vi "FPGAController_v4.vi"() -> ()   [LabVIEW 2015]
uses:
  <vilib>/Utility/miscctls.llb/LVPointTypeDef.ctl
  <vilib>/FPGAPlugInAG/PXIe-7971R/niLvFpga_Open_PXIe-7971R.vi
  <vilib>/Utility/error.llb/Error Cluster From Error Code.vi
  <vilib>/rvi/errors/niLvFpgaAdjustHostInterfaceError.vi
  <userlib>/_OpenG.lib/comparison/comparison.llb/DBL Changed__ogtk.vi
  <userlib>/_OpenG.lib/file/file.llb/Strip Path Extension - Path__ogtk.vi
  <userlib>/_OpenG.lib/comparison/comparison.llb/Boolean Changed__ogtk.vi
  <vilib>/addons/database/Connection.llb/Conn Execute.vi
  <vilib>/addons/database/Recordset.llb/Rec Fetch Recordset Data (R).vi
  <vilib>/addons/database/Recordset.llb/Rec Destroy - Connection.vi
  <vilib>/FPGAPlugInAG/PXIe-7971R/niLvFpga_Close_PXIe-7971R.vi
  <vilib>/rvi/interface/nirviOpenFPGA/nirviOpenFPGA.xnode
  FPGA Bitfiles/FPGAnew_FPGATarget_FPGAcode5762_R0izv7IQhAo.lvbitx
  <vilib>/rvi/interface/nirviReadWriteControl/nirviReadWriteControl.xnode
  <vilib>/rvi/interface/nirviMethod/nirviMethod.xnode
  <vilib>/FPGA/interface/niFpgaViExecutionMode.ctl
  <vilib>/addons/database/_DB Variant To Data/Database Variant To Data.xnode
  <vilib>/rvi/interface/nirviCloseFPGA/nirviCloseFPGA.xnode
  <vilib>/addons/database/NI_Database_API.lvlib
  NiFpgaLv.dll
panel:
  out "Time Betwee Shots":dbl
  in  "Min. Time\nBetween Shots (s)":dbl
  in  "Rate Limiting":bool
  out "Update Threshold":bool
  in  "Auto Threshold":bool
  in  "stop":bool
  out "stopping":bool
  in  "One Shot Mode":bool
  out "High Velocity":dbl=100000.0
  out "Low Velocity":dbl=1000.0
  out "Low velocity count":i32=21000
  out "High velocity count":i32=210
  out "Filter 1 Peak":i32=295996
  out "Filter 2 Peak":i32=120664
  out "Filter 3 Peak":i32=46254
  out "Filter 4 Peak":i32=18191
  out "Filter 5 Peak":i32=13910
  out "Filter 6 Peak":i32=9863
  out "Filter 7 Peak":i32=7483
  in  "Zero Peak Values":bool
  in  "Peak-Threshold Factor":dbl=2.0
  in  "Assign Threshold":bool
  in  "Filter1 Threshold":i32=-887988
  in  "Filter2 Threshold":i32=-361992
  in  "Filter3 Threshold":i32=-138762
  in  "Filter4 Threshold":i32=-54306
  in  "Filter5 Threshold":i32=-41730
  in  "Filter6 Threshold":i32=-29358
  in  "Filter7 Threshold":i32=-21165
  out "High Charge Limit (fC)":dbl=100.0
  out "Low Charge Limit (fC)":dbl
  out "High Charge Limit":i16
  out "Low Charge Limit":i16
  out "Low Mass (kg)":dbl
  out "High Mass (kg)":dbl=inf
  out "Peletron (MV)":dbl=2.0
  in  "Run Mode":bool
  out "High Mass Limit":fxp<+,31,17>
  out "Low Mass Limit":fxp<+,31,17>
  out "error out":errorcluster
  out "Sensitivity":dbl
  out "Last Update:":timestamp
  out "Updating FPGA":bool
  in  "Delay Ring":dbl(ring)=3.15039 items=["Custom"]
  in  "Delay Value":dbl=3.0 min=0.0
  in  "Delay Name":string
  in  "Rearm Trigger":bool
  out "Armed":bool
  in  "Add Delay":bool
  in  "Raise Threshold":bool
  in  "Lower Threshold":bool
  out "Del Armed":bool
  # "Dubugging"
  # "Settings"
  # "Thresholds"
  # "Peaks"
  # "Independent Variable"
  # "Threshold 1"
  # "Peak 1"
  # "Low Vel."
  # "High Vel."
  # "Threshold 2"
  # "Peak 2"
  # "Low Q (fC)"
  # "High Q (fC)"
  # "Plate Control While Loop Counter"
  # "Threshold 3"
  # "Peak 3"
  # "Low Mass (kg)"
  # "High Q (fC)"
  # "Threshold 4"
  # "Peak 4"
  # "Sens. (V/pC)"
  # "Peletron (MV)"
  # "Current Value of Running Average"
  # "Threshold 5"
  # "Peak 5"
  # "Peak Threshold Factor"
  # "Threshold 6"
  # "Peak 6"
  # "Delay Trigger"
  # "Dist. from 2nd Det. (m)"
  # "Name"
  # "Threshold 7"
  # "Peak 7"
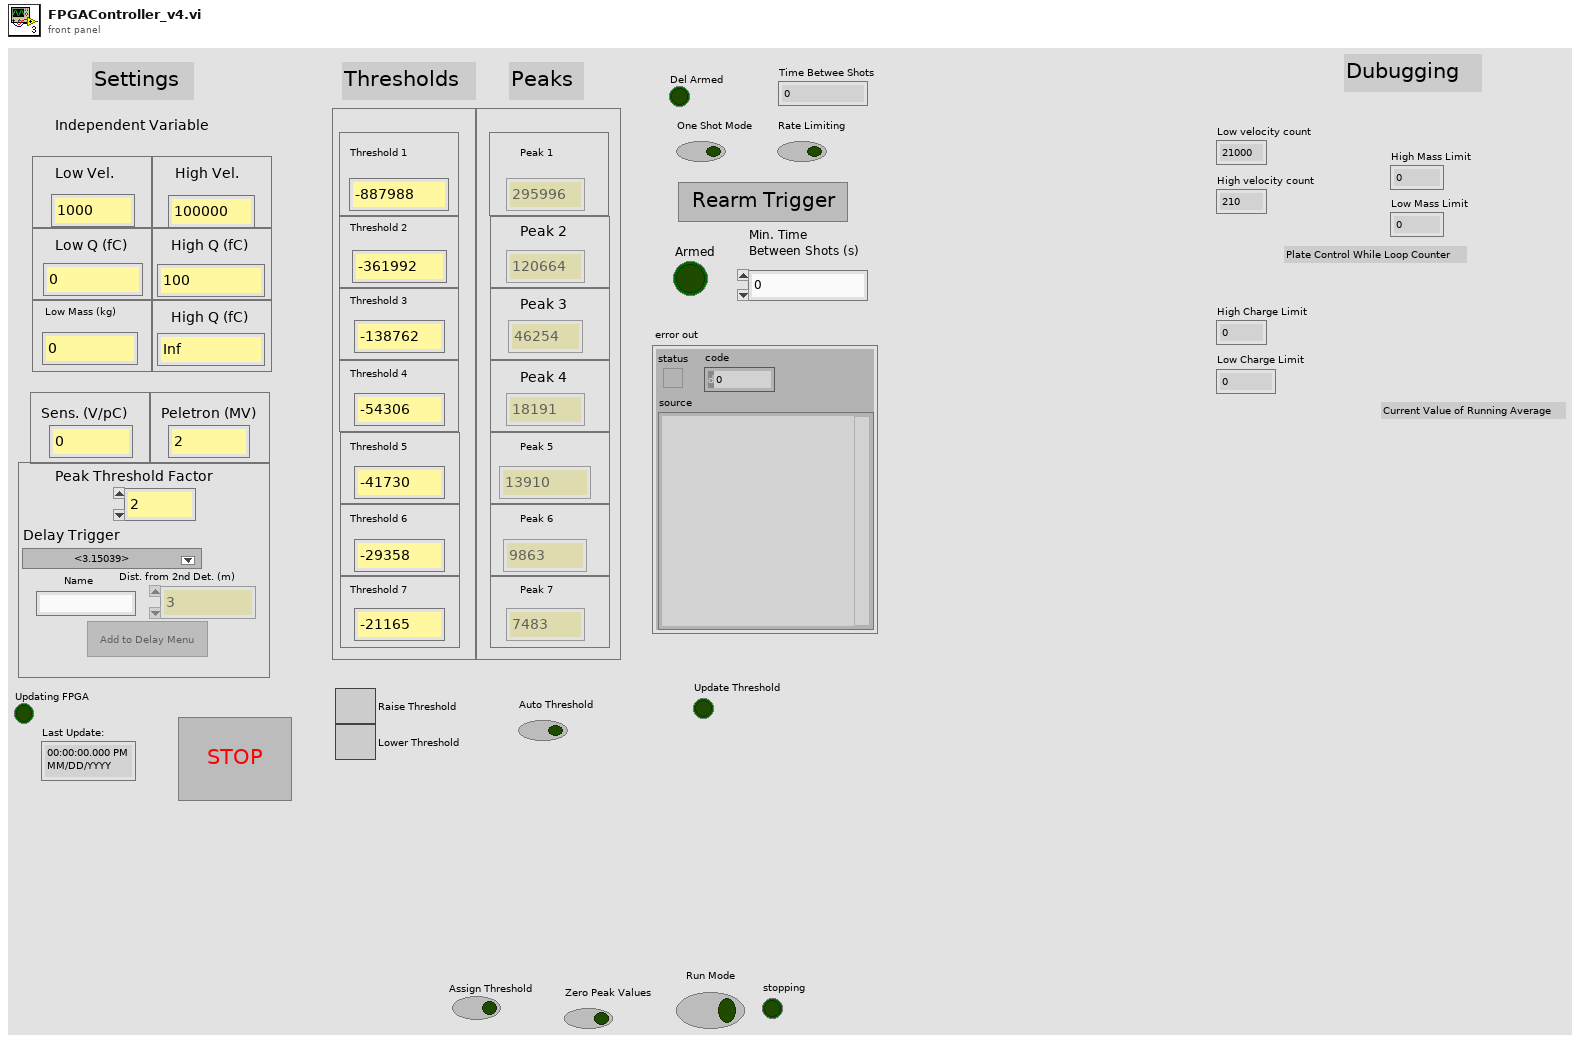
[diagram p1: front panel]
types:
  T1 = typedef "LVPointTypeDef.ctl" = cluster{"Horizontal":i16, "Vertical":i16}
  T2 = enum8{"Enabled", "Disabled", "Disabled and Grayed Out"}
  T3 = typedef "NI_Database_API.lvlib/Conn ObjectReference.ctl" = refnum<k1>
  T4 = cluster{"Filter 1 Peak":i32, "Filter 2 Peak":i32, "Filter 3 Peak":i32, "Filter 4 Peak":i32, "Filter 5 Peak":i32, "Filter 6 Peak":i32, "Filter 7 Peak":i32}
  T5 = typedef "NI_Database_API.lvlib/Rec ObjectReference.ctl" = refnum<k1>
  T6 = typedef "LVStringsAndValuesArrayTypeDef_DBL.ctl" = cluster{"String":string, "Value":dbl}[]
  T7 = cluster{"Numeric":dbl, "Numeric":dbl, "Numeric":dbl, "Numeric":dbl, "Numeric":dbl, "Numeric":dbl, i32, dbl, "Value":dbl, fxp<+,16,7>, bool}
  T8 = cluster{"Low Velocity Count":i32, "High Velocity Count":i32, "Low Charge Limit (ADC ticks)":i16, "High Charge Limit (ADC ticks)":i16, "Low Mass (ADC*cycle^2)":i64, "High Mass (ADC*cycle^2)":i64, "Mult":fxp<+,16,7>, "Mult Use?":bool}
  T9 = cluster{"Filter 1 Detector 3 Correlation":i32, "Filter 2 Detector 3 Correlation":i32, "Filter 3 Detector 3 Correlation":i32, "Filter 4 Detector 3 Correlation":i32, "Filter 5 Detector 3 Correlation":i32, "Filter 6 Detector 3 Correlation":i32, "Filter 7 Detector 3 Correlation":i32}
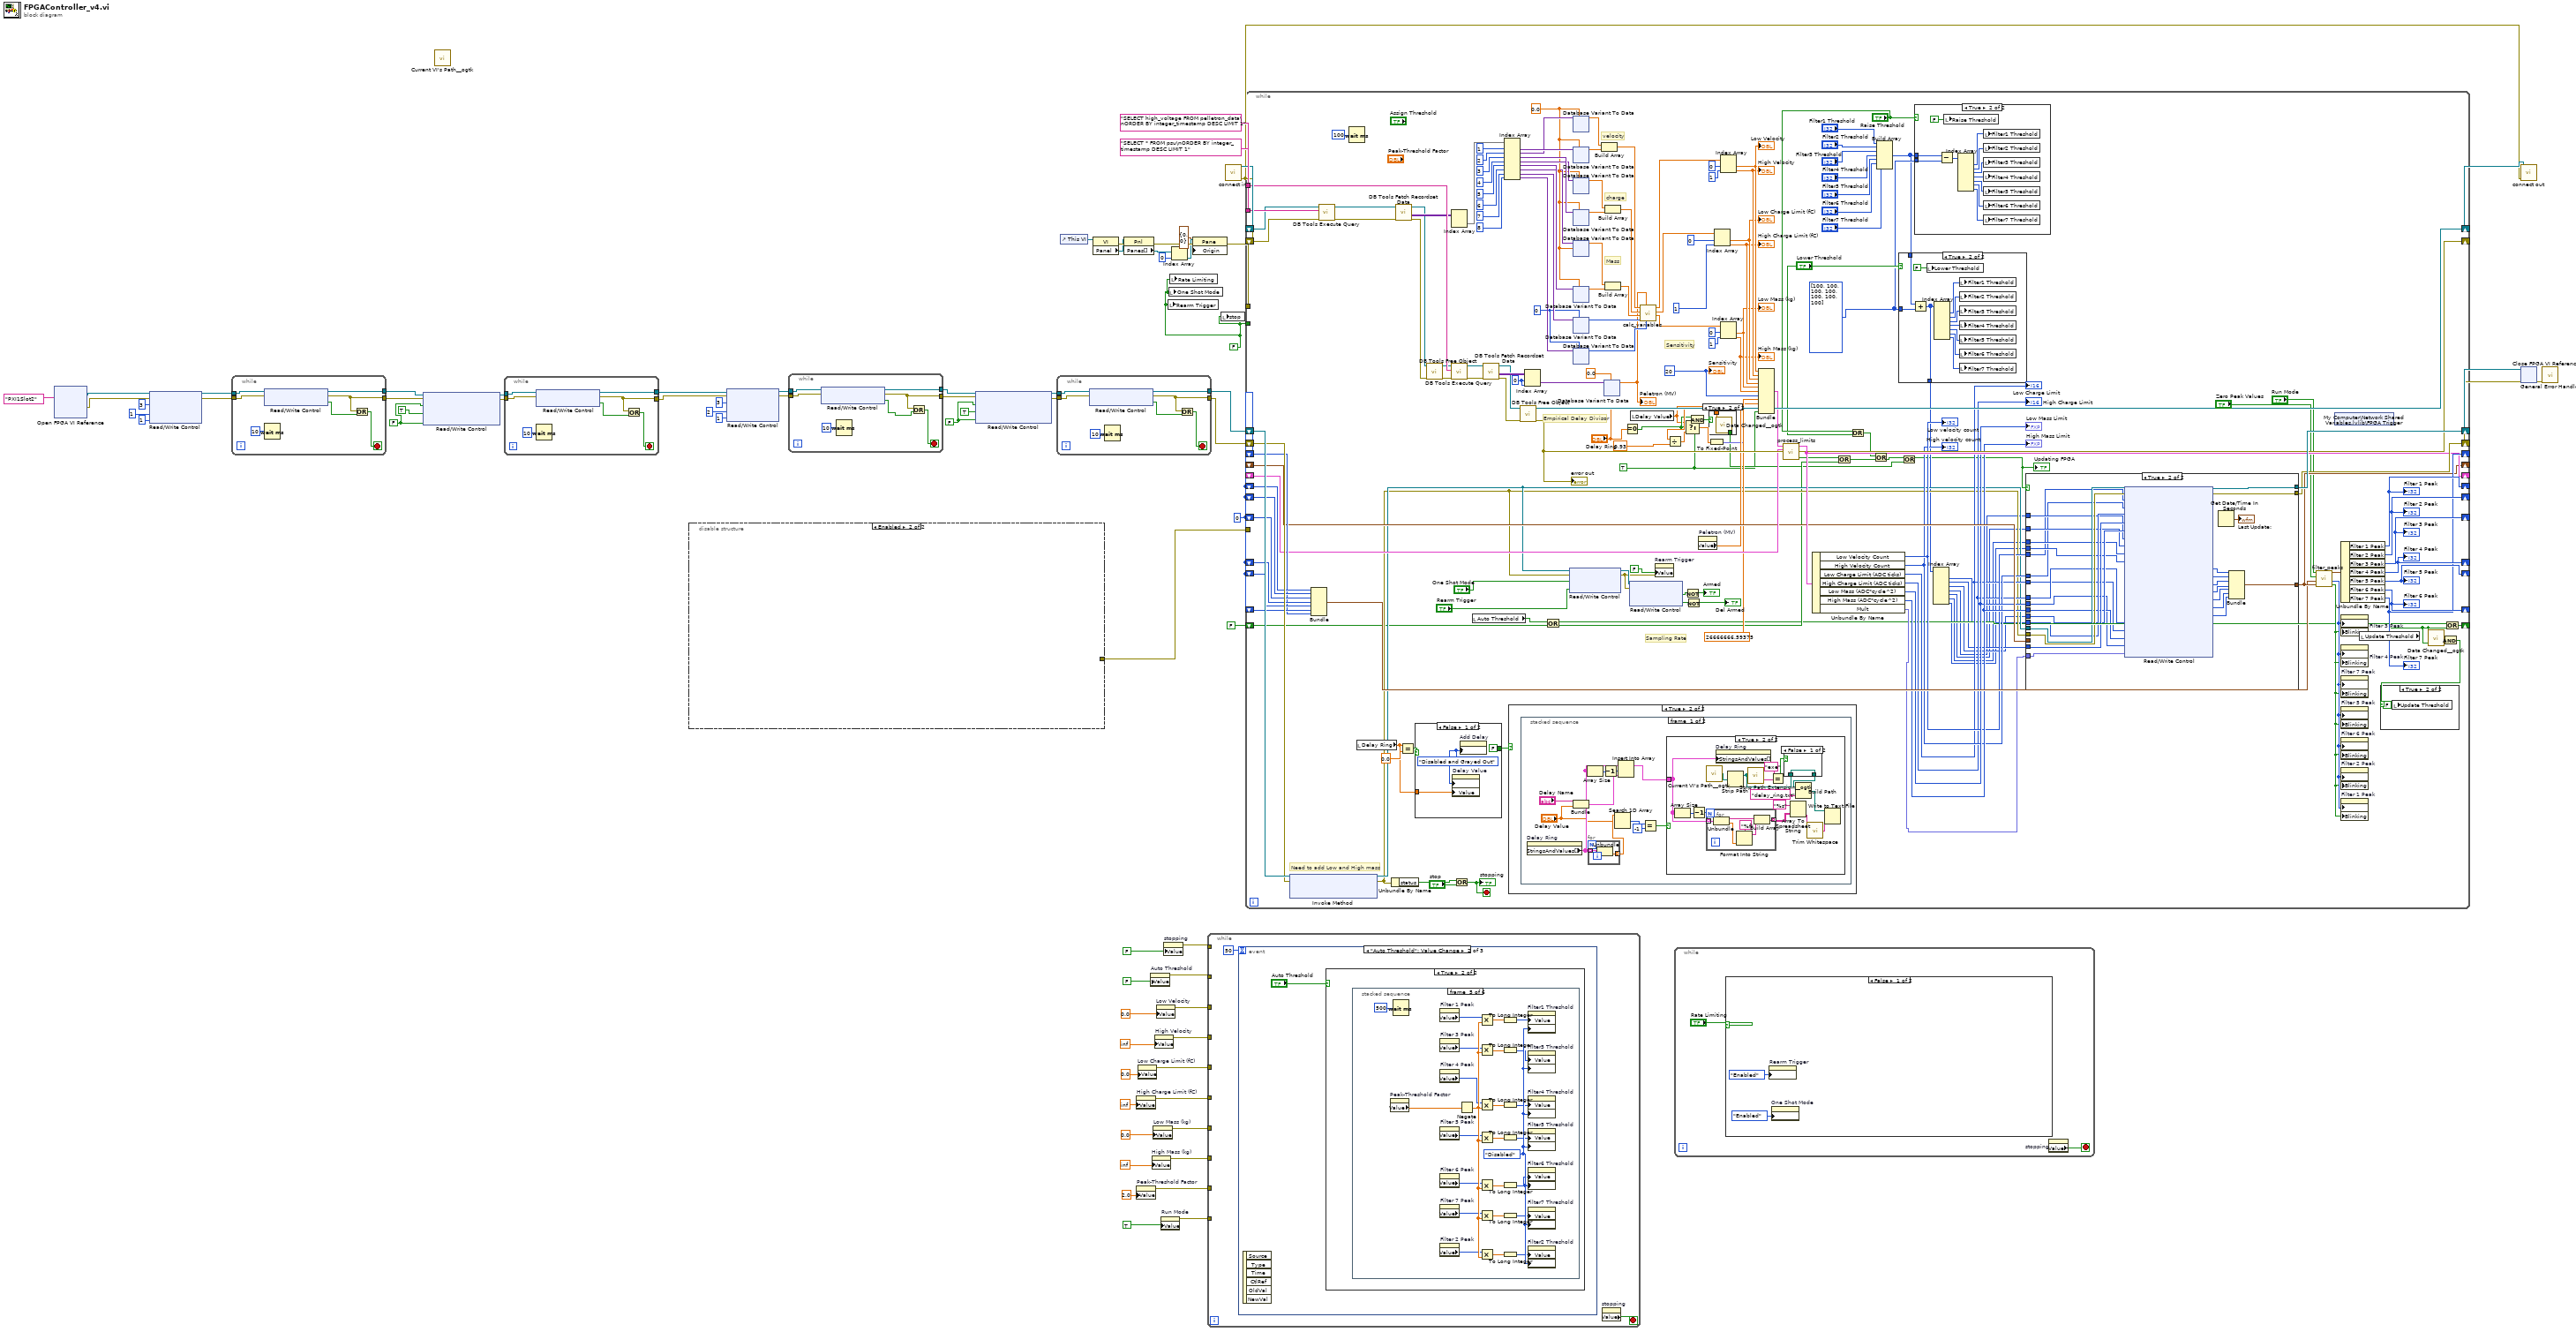
[diagram p0: block diagram]
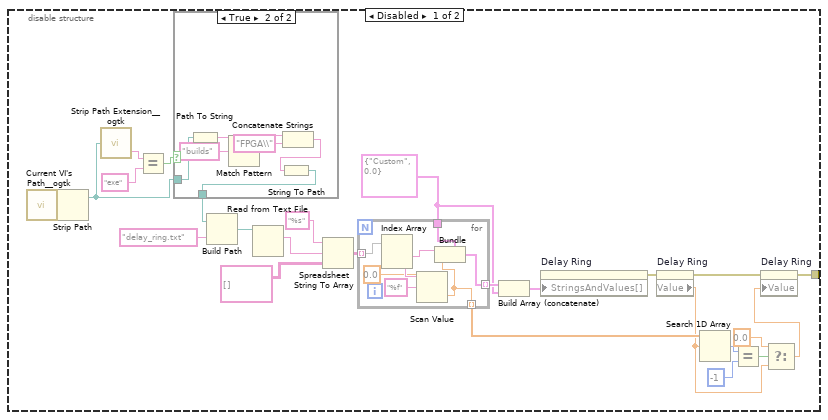
[diagram p2: hidden frame]
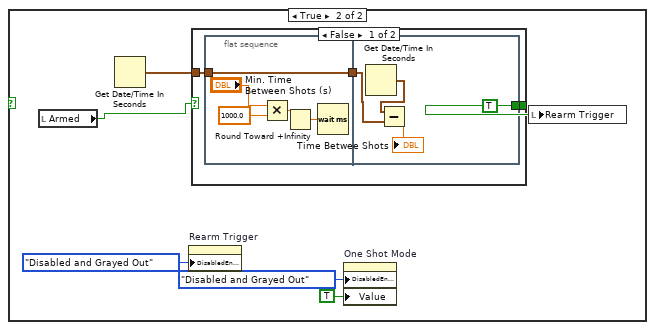
[diagram p4: hidden frame]
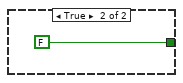
[diagram p5: hidden frame]
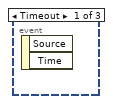
[diagram p6: hidden frame]
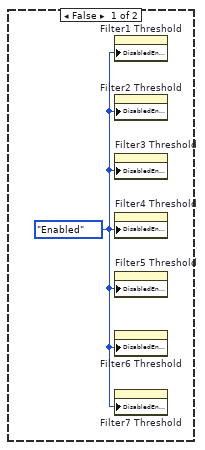
[diagram p7: hidden frame]
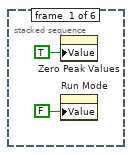
[diagram p8: hidden frame]
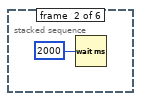
[diagram p9: hidden frame]
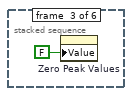
[diagram p10: hidden frame]
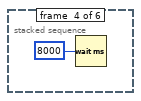
[diagram p11: hidden frame]
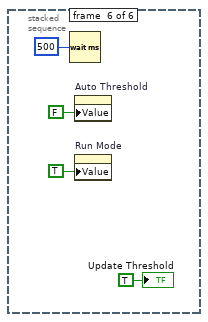
[diagram p12: hidden frame]
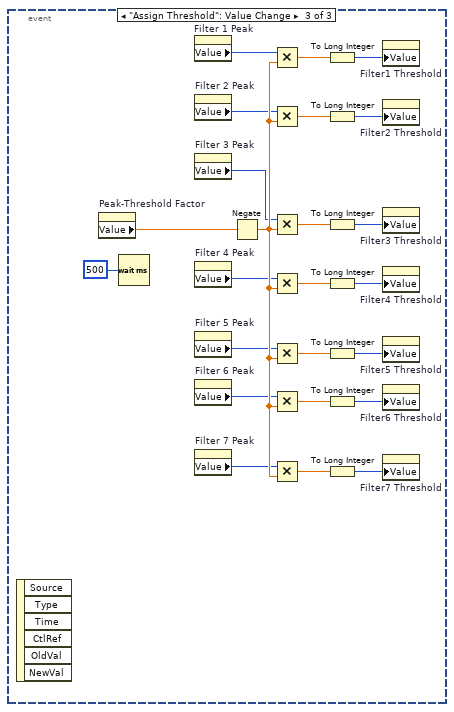
[diagram p13: hidden frame]
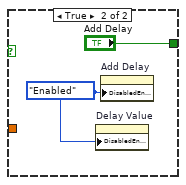
[diagram p18: hidden frame]
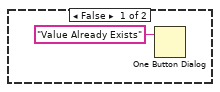
[diagram p20: hidden frame]
diagram:
  w6 = FALSE ("User Command Commit")
  w7 = FALSE ("User Command Commit")
  w29 = FALSE
  w69 = 0
  n1 = xnode "Open FPGA VI Reference"("resource name"=tag "PXI1Slot2") -> ("FPGA VI Reference Out"=w4:refnum<k20>, "error out"=w3:errorcluster)  [unwired: 1 in]
  n2 = xnode "Read/Write Control"("FPGA VI Reference In"=w4, "error in"=w3, "User Command"=u8 3, "User Data 0"=u8 1, "User Data 1"=u8 1) -> ("FPGA VI Reference Out"=w25:refnum<k20>, "error out"=w24:errorcluster)
  n3 = while {
    tunnel: w25 -> [w77]
    tunnel: w24 -> [w76]
    tunnel: [w75] -> w11
    tunnel: [w73] -> w12
    stop <- w74 stop-if-true
    n4 = xnode "Read/Write Control"("FPGA VI Reference In"=w77, "error in"=w76) -> ("FPGA VI Reference Out"=w73:refnum<k20>, "error out"=w75:errorcluster, "User Command Idle"=w71:bool)
    n5 = Wait (ms)(milliseconds to wait=u32 10) -> ()  [unwired: 1 out]
    n6 = Or(x=w75, y=w71) -> (x .or. y?=w74:bool)
  }
  n7 = xnode "Read/Write Control"("FPGA VI Reference In"=w12, "error in"=w11, "User Command Commit"=w7, "User Command Commit"=TRUE, "User Command Commit"=w7) -> ("FPGA VI Reference Out"=w14:refnum<k20>, "error out"=w13:errorcluster)
  n8 = call <userlib>:"Current VI's Path__ogtk.vi"() -> ()  [unwired: 1 in, 1 out]
  n9 = while {
    tunnel: w14 -> [w84]
    tunnel: w13 -> [w83]
    tunnel: [w82] -> w9
    tunnel: [w80] -> w10
    stop <- w81 stop-if-true
    n10 = xnode "Read/Write Control"("FPGA VI Reference In"=w84, "error in"=w83) -> ("FPGA VI Reference Out"=w80:refnum<k20>, "error out"=w82:errorcluster, "User Command Idle"=w78:bool)
    n11 = Wait (ms)(milliseconds to wait=u32 10) -> ()  [unwired: 1 out]
    n12 = Or(x=w82, y=w78) -> (x .or. y?=w81:bool)
  }
  n13 = disable-structure shown="Enabled" {
    disable-tunnel: [w91 _] -> w31
    frame Disabled {
      w100 = cluster{"String":string, "Value":dbl} {"String"="Custom", "Value"=0.0}
      n14 = call <userlib>:"Current VI's Path__ogtk.vi"() -> ("Current VI's Path (+ Relative)"=w109:path)  [unwired: 1 in]
      n15 = Strip Path(path=w109) -> (stripped path=w95:path)  [unwired: 1 out]
      n16 = call-poly <userlib>:"Strip Path Extension__ogtk.vi"("path"=w95) -> ("extension"=w99:string)  [unwired: 1 out]
      n17 = Equal?(x=w99, y="exe") -> (x = y?=w96:bool)
      n18 = case shown="True" w96 {
        tunnel: w95 -> [w118 w125]
        tunnel: [w118 w119] -> w94
        frame False {
        }
        frame True {
          n19 = Path To String(path=w125) -> (string=w124:string)
          n20 = Match Pattern(string=w124, regular expression="builds") -> (before substring=w122:string)  [unwired: 1 in, 3 out]
          n21 = Concatenate Strings(w122, "FPGA\\" ("string")) -> (w120:string)
          n22 = String To Path(string=w120) -> (path=w119:path)
        }
      }
      n23 = Build Path(base path=w94, name or relative path="delay_ring.txt") -> (appended path=w97:path)
      n24 = Read from Text File(file (use dialog)=w97) -> (text=w107:string)  [unwired: 3 in, 3 out]
      n25 = Spreadsheet String To Array(format string="%s", spreadsheet string=w107, array type (2D Dbl)=string[][] []) -> (array=w104:string[][])  [unwired: 1 in]
      n26 = for {
        tunnel: w104 -> [w117] mode=indexing
        tunnel: w100 -> [w115]
        tunnel: [w111] -> w101 mode=indexing
        tunnel: [w110] -> w93 mode=indexing
        n27 = Index Array(array=w117) -> (element #1=w116:string, element #2=w114:string)  [unwired: 2 in]
        n28 = Scan Value(string=w114, format string="%f", default (0 dbl)=0.0) -> (value=w110:dbl)  [unwired: 1 out]
        n29 = Bundle(cluster=w115, "String"=w116, "Value"=w110) -> (w111:cluster{"String":string, "Value":dbl})
      }
      n30 = Build Array (concatenate)(w101, w100) -> (w103:cluster{"String":string, "Value":dbl}[])
      n31 = property on="Delay Ring" class="Ring (strict)"("StringsAndValues[]"=w103) -> (error out=w102:errorcluster)  [unwired: 2 in, 1 out]
      n32 = property on="Delay Ring" class="Ring (strict)"(error in=w102) -> (error out=w92:errorcluster, "Value"=w86:dbl)  [unwired: 1 in, 1 out]
      n33 = Search 1D Array(1D array=w93, element=w86) -> (index of element=w90:i32)  [unwired: 1 in]
      n34 = Equal?(x=w90, y=-1) -> (x = y?=w88:bool)
      n35 = Select(t=0.0, s=w88, f=w86) -> (s? t:f=w87:dbl)
      n36 = property on="Delay Ring" class="Ring (strict)"(error in=w92, "Value"=w87) -> (error out=w91:errorcluster)  [unwired: 1 in, 1 out]
    }
    frame Enabled {
    }
  }
  n37 = xnode "Read/Write Control"("FPGA VI Reference In"=w10, "error in"=w9, "User Command"=u8 3, "User Data 0"=u8 2, "User Data 1"=u8 1) -> ("FPGA VI Reference Out"=w20:refnum<k20>, "error out"=w19:errorcluster)
  n38 = while {
    tunnel: w20 -> [w132]
    tunnel: w19 -> [w131]
    tunnel: [w130] -> w17
    tunnel: [w128] -> w18
    stop <- w129 stop-if-true
    n39 = xnode "Read/Write Control"("FPGA VI Reference In"=w132, "error in"=w131) -> ("FPGA VI Reference Out"=w128:refnum<k20>, "error out"=w130:errorcluster, "User Command Idle"=w126:bool)
    n40 = Wait (ms)(milliseconds to wait=u32 10) -> ()  [unwired: 1 out]
    n41 = Or(x=w130, y=w126) -> (x .or. y?=w129:bool)
  }
  n42 = xnode "Read/Write Control"("FPGA VI Reference In"=w18, "error in"=w17, "User Command Commit"=w6, "User Command Commit"=TRUE, "User Command Commit"=w6) -> ("FPGA VI Reference Out"=w16:refnum<k20>, "error out"=w15:errorcluster)
  n43 = while {
    tunnel: w16 -> [w139]
    tunnel: w15 -> [w138]
    tunnel: [w137] -> w2
    tunnel: [w135] -> w1
    stop <- w136 stop-if-true
    n44 = xnode "Read/Write Control"("FPGA VI Reference In"=w139, "error in"=w138) -> ("FPGA VI Reference Out"=w135:refnum<k20>, "error out"=w137:errorcluster, "User Command Idle"=w133:bool)
    n45 = Wait (ms)(milliseconds to wait=u32 10) -> ()  [unwired: 1 out]
    n46 = Or(x=w137, y=w133) -> (x .or. y?=w136:bool)
  }
  n47 = control-ref of="This VI"() -> (w41:refnum<vi>)
  n48 = property class="VI"(reference=w41) -> (error out=w40:errorcluster, "Panel"=w39:refnum<vi>)  [unwired: 1 in, 1 out]
  n49 = property class="Pnl"(reference=w39, error in=w40) -> (error out=w38:errorcluster, "Panes[]"=w37:refnum<vi>[])  [unwired: 1 out]
  n50 = property on="High Charge Limit (fC)" class="DigNum (strict)"("Value"=inf ("High Charge Limit (fC)")) -> (error out=w56:errorcluster)  [unwired: 2 in, 1 out]
  n51 = property on="Peak-Threshold Factor" class="DigNum (strict)"("Value"=2.0 ("Peak-Threshold Factor")) -> (error out=w50:errorcluster)  [unwired: 2 in, 1 out]
  n52 = property on="Low Charge Limit (fC)" class="DigNum (strict)"("Value"=0.0 ("Low Charge Limit (fC)")) -> (error out=w58:errorcluster)  [unwired: 2 in, 1 out]
  n53 = property on="Auto Threshold" class="Bool (strict)"("Value"=FALSE ("Auto Threshold")) -> (error out=w64:errorcluster)  [unwired: 2 in, 1 out]
  n54 = property on="High Mass (kg)" class="DigNum (strict)"("Value"=inf ("High Mass (kg)")) -> (error out=w52:errorcluster)  [unwired: 2 in, 1 out]
  n55 = property on="Low Mass (kg)" class="DigNum (strict)"("Value"=0.0 ("Low Mass (kg)")) -> (error out=w54:errorcluster)  [unwired: 2 in, 1 out]
  n56 = property on="High Velocity" class="DigNum (strict)"("Value"=inf ("High Velocity")) -> (error out=w60:errorcluster)  [unwired: 2 in, 1 out]
  n57 = property on="Low Velocity" class="DigNum (strict)"("Value"=0.0 ("Low Velocity")) -> (error out=w62:errorcluster)  [unwired: 2 in, 1 out]
  n58 = property on="Run Mode" class="Bool (strict)"("Value"=TRUE ("Run Mode")) -> (error out=w48:errorcluster)  [unwired: 2 in, 1 out]
  n59 = property on="stopping" class="Bool (strict)"("Value"=FALSE ("stopping")) -> (error out=w66:errorcluster)  [unwired: 2 in, 1 out]
  n60 = local write "Rearm Trigger"(w29) -> ()
  n61 = local write "One Shot Mode"(w29) -> ()
  n62 = local write "Rate Limiting"(w29) -> ()
  n63 = Index Array(array=w37, index=0) -> (element=w35:refnum<vi>)
  n64 = property class="Pane"(reference=w35, error in=w38, "Origin"=T1 {"Horizontal"=0, "Vertical"=0}) -> (error out=w33:errorcluster)  [unwired: 1 out]
  n65 = while {
    tunnel: w66 -> [_]
    tunnel: w64 -> [_]
    tunnel: w62 -> [_]
    tunnel: w60 -> [_]
    tunnel: w58 -> [_]
    tunnel: w56 -> [_]
    tunnel: w54 -> [_]
    tunnel: w52 -> [_]
    tunnel: w50 -> [_]
    tunnel: w48 -> [_]
    stop <- w141 stop-if-true
    n66 = event shown="[1] \"Auto Threshold\": Value Change" {
      selector: _ -> [_ _ _]
      dyn-events: _ -> [_ _ _]
      timeout: 50 -> [_ _ _]
      event Timeout {
        n67 = event-data() -> ()  [unwired: 1 in, 2 out]
      }
      event "Auto Threshold": Value Change {
        n68 = event-data() -> ()  [unwired: 1 in, 6 out]
        n69 = case shown="True" "Auto Threshold" {
          frame False {
            w143 = T2."Enabled" ("Disabled")
            n70 = property on="Filter1 Threshold" class="DigNum (strict)"("DisabledEnum"=w143) -> ()  [unwired: 2 in, 2 out]
            n71 = property on="Filter2 Threshold" class="DigNum (strict)"("DisabledEnum"=w143) -> ()  [unwired: 2 in, 2 out]
            n72 = property on="Filter3 Threshold" class="DigNum (strict)"("DisabledEnum"=w143) -> ()  [unwired: 2 in, 2 out]
            n73 = property on="Filter4 Threshold" class="DigNum (strict)"("DisabledEnum"=w143) -> ()  [unwired: 2 in, 2 out]
            n74 = property on="Filter5 Threshold" class="DigNum (strict)"("DisabledEnum"=w143) -> ()  [unwired: 2 in, 2 out]
            n75 = property on="Filter6 Threshold" class="DigNum (strict)"("DisabledEnum"=w143) -> ()  [unwired: 2 in, 2 out]
            n76 = property on="Filter7 Threshold" class="DigNum (strict)"("DisabledEnum"=w143) -> ()  [unwired: 2 in, 2 out]
          }
          frame True {
            n77 = stacked-sequence {
              frame #0 {
                n78 = property on="Zero Peak Values" class="Bool (strict)"("Value"=TRUE ("Zero Peak Values")) -> ()  [unwired: 2 in, 2 out]
                n79 = property on="Run Mode" class="Bool (strict)"("Value"=FALSE ("Run Mode")) -> ()  [unwired: 2 in, 2 out]
              }
              frame #1 {
                n80 = Wait (ms)(milliseconds to wait=u32 2000) -> ()  [unwired: 1 out]
              }
              frame #2 {
                n81 = property on="Zero Peak Values" class="Bool (strict)"("Value"=FALSE ("Zero Peak Values")) -> ()  [unwired: 2 in, 2 out]
              }
              frame #3 {
                n82 = Wait (ms)(milliseconds to wait=u32 8000) -> ()  [unwired: 1 out]
              }
              frame #4 {
                w173 = T2."Disabled" ("Disabled")
                n83 = property on="Peak-Threshold Factor" class="DigNum (strict)"() -> ("Value"=w158:dbl)  [unwired: 2 in, 2 out]
                n84 = Wait (ms)(milliseconds to wait=u32 500) -> ()  [unwired: 1 out]
                n85 = property on="Filter 1 Peak" class="DigNum (strict)"() -> ("Value"=w156:i32)  [unwired: 2 in, 2 out]
                n86 = property on="Filter 3 Peak" class="DigNum (strict)"() -> ("Value"=w154:i32)  [unwired: 2 in, 2 out]
                n87 = property on="Filter 4 Peak" class="DigNum (strict)"() -> ("Value"=w153:i32)  [unwired: 2 in, 2 out]
                n88 = property on="Filter 5 Peak" class="DigNum (strict)"() -> ("Value"=w152:i32)  [unwired: 2 in, 2 out]
                n89 = property on="Filter 6 Peak" class="DigNum (strict)"() -> ("Value"=w151:i32)  [unwired: 2 in, 2 out]
                n90 = property on="Filter 7 Peak" class="DigNum (strict)"() -> ("Value"=w150:i32)  [unwired: 2 in, 2 out]
                n91 = property on="Filter 2 Peak" class="DigNum (strict)"() -> ("Value"=w155:i32)  [unwired: 2 in, 2 out]
                n92 = Negate(x=w158) -> (-x=w157:dbl)
                n93 = Multiply(x=w156, y=w157) -> (x*y=w172:dbl)
                n94 = Multiply(x=w154, y=w157) -> (x*y=w168:dbl)
                n95 = Multiply(x=w153, y=w157) -> (x*y=w166:dbl)
                n96 = Multiply(x=w152, y=w157) -> (x*y=w164:dbl)
                n97 = Multiply(x=w151, y=w157) -> (x*y=w162:dbl)
                n98 = Multiply(x=w150, y=w157) -> (x*y=w160:dbl)
                n99 = Multiply(x=w155, y=w157) -> (x*y=w170:dbl)
                n100 = To Long Integer(number=w172) -> (32bit integer=w171:i32)
                n101 = To Long Integer(number=w168) -> (32bit integer=w167:i32)
                n102 = To Long Integer(number=w166) -> (32bit integer=w165:i32)
                n103 = To Long Integer(number=w164) -> (32bit integer=w163:i32)
                n104 = To Long Integer(number=w162) -> (32bit integer=w161:i32)
                n105 = To Long Integer(number=w160) -> (32bit integer=w159:i32)
                n106 = To Long Integer(number=w170) -> (32bit integer=w169:i32)
                n107 = property on="Filter1 Threshold" class="DigNum (strict)"("Value"=w171, "DisabledEnum"=w173) -> ()  [unwired: 2 in, 2 out]
                n108 = property on="Filter3 Threshold" class="DigNum (strict)"("Value"=w167, "DisabledEnum"=w173) -> ()  [unwired: 2 in, 2 out]
                n109 = property on="Filter4 Threshold" class="DigNum (strict)"("Value"=w165, "DisabledEnum"=w173) -> ()  [unwired: 2 in, 2 out]
                n110 = property on="Filter5 Threshold" class="DigNum (strict)"("Value"=w163, "DisabledEnum"=w173) -> ()  [unwired: 2 in, 2 out]
                n111 = property on="Filter6 Threshold" class="DigNum (strict)"("Value"=w161, "DisabledEnum"=w173) -> ()  [unwired: 2 in, 2 out]
                n112 = property on="Filter7 Threshold" class="DigNum (strict)"("Value"=w159, "DisabledEnum"=w173) -> ()  [unwired: 2 in, 2 out]
                n113 = property on="Filter2 Threshold" class="DigNum (strict)"("Value"=w169, "DisabledEnum"=w173) -> ()  [unwired: 2 in, 2 out]
              }
              frame #5 {
                n114 = Wait (ms)(milliseconds to wait=u32 500) -> ()  [unwired: 1 out]
                n115 = property on="Auto Threshold" class="Bool (strict)"("Value"=FALSE ("Auto Threshold")) -> ()  [unwired: 2 in, 2 out]
                n116 = property on="Run Mode" class="Bool (strict)"("Value"=TRUE ("Run Mode")) -> ()  [unwired: 2 in, 2 out]
                "Update Threshold" <- TRUE ("Update Threshold")
              }
            }
          }
        }
      }
      event "Assign Threshold": Value Change {
        n117 = event-data() -> ()  [unwired: 1 in, 6 out]
        n118 = property on="Peak-Threshold Factor" class="DigNum (strict)"() -> ("Value"=w192:dbl)  [unwired: 2 in, 2 out]
        n119 = Wait (ms)(milliseconds to wait=u32 500) -> ()  [unwired: 1 out]
        n120 = property on="Filter 1 Peak" class="DigNum (strict)"() -> ("Value"=w191:i32)  [unwired: 2 in, 2 out]
        n121 = property on="Filter 2 Peak" class="DigNum (strict)"() -> ("Value"=w190:i32)  [unwired: 2 in, 2 out]
        n122 = property on="Filter 3 Peak" class="DigNum (strict)"() -> ("Value"=w189:i32)  [unwired: 2 in, 2 out]
        n123 = property on="Filter 4 Peak" class="DigNum (strict)"() -> ("Value"=w188:i32)  [unwired: 2 in, 2 out]
        n124 = property on="Filter 5 Peak" class="DigNum (strict)"() -> ("Value"=w187:i32)  [unwired: 2 in, 2 out]
        n125 = property on="Filter 6 Peak" class="DigNum (strict)"() -> ("Value"=w186:i32)  [unwired: 2 in, 2 out]
        n126 = property on="Filter 7 Peak" class="DigNum (strict)"() -> ("Value"=w185:i32)  [unwired: 2 in, 2 out]
        n127 = Negate(x=w192) -> (-x=w194:dbl)
        n128 = Multiply(x=w191, y=w194) -> (x*y=w201:dbl)
        n129 = Multiply(x=w190, y=w194) -> (x*y=w199:dbl)
        n130 = Multiply(x=w189, y=w194) -> (x*y=w198:dbl)
        n131 = Multiply(x=w188, y=w194) -> (x*y=w197:dbl)
        n132 = Multiply(x=w187, y=w194) -> (x*y=w196:dbl)
        n133 = Multiply(x=w186, y=w194) -> (x*y=w195:dbl)
        n134 = Multiply(x=w185, y=w194) -> (x*y=w200:dbl)
        n135 = To Long Integer(number=w201) -> (32bit integer=w184:i32)
        n136 = To Long Integer(number=w199) -> (32bit integer=w183:i32)
        n137 = To Long Integer(number=w198) -> (32bit integer=w182:i32)
        n138 = To Long Integer(number=w197) -> (32bit integer=w181:i32)
        n139 = To Long Integer(number=w196) -> (32bit integer=w180:i32)
        n140 = To Long Integer(number=w195) -> (32bit integer=w179:i32)
        n141 = To Long Integer(number=w200) -> (32bit integer=w178:i32)
        n142 = property on="Filter1 Threshold" class="DigNum (strict)"("Value"=w184) -> ()  [unwired: 2 in, 2 out]
        n143 = property on="Filter2 Threshold" class="DigNum (strict)"("Value"=w183) -> ()  [unwired: 2 in, 2 out]
        n144 = property on="Filter3 Threshold" class="DigNum (strict)"("Value"=w182) -> ()  [unwired: 2 in, 2 out]
        n145 = property on="Filter4 Threshold" class="DigNum (strict)"("Value"=w181) -> ()  [unwired: 2 in, 2 out]
        n146 = property on="Filter5 Threshold" class="DigNum (strict)"("Value"=w180) -> ()  [unwired: 2 in, 2 out]
        n147 = property on="Filter6 Threshold" class="DigNum (strict)"("Value"=w179) -> ()  [unwired: 2 in, 2 out]
        n148 = property on="Filter7 Threshold" class="DigNum (strict)"("Value"=w178) -> ()  [unwired: 2 in, 2 out]
      }
    }
    n149 = property on="stopping" class="Bool (strict)"() -> ("Value"=w141:bool)  [unwired: 2 in, 2 out]
  }
  n150 = local write "stop"(w29) -> ()
  n151 = call "connect in.vi"() -> ("error out"=w42:errorcluster, "Database Connection"=w43:T3)  [unwired: 7 in, 1 out]
  n152 = while {
    shift-right: [w363] -> w68
    shift-left: w1 -> [w367]
    shift-right: [w362] -> w67
    shift-left: w2 -> [w366]
    shift-right: [w358] -> _
    shift-left: w69 -> [w351]
    shift-right: [w357] -> _
    shift-left: w69 -> [w350]
    shift-right: [w356] -> _
    shift-left: w69 -> [w349]
    shift-right: [w355] -> _
    shift-left: w69 -> [w348]
    shift-right: [w354] -> _
    shift-left: w69 -> [w347]
    shift-right: [w360] -> _
    shift-left: w69 -> [w353]
    shift-right: [w359] -> _
    shift-left: w69 -> [w352]
    tunnel: "SELECT * FROM psu\nORDER BY integer_timestamp DESC LIMIT 1" ("SQL query") -> [w346]
    tunnel: "SELECT high_voltage FROM pelletron_data\nORDER BY integer_timestamp DESC LIMIT 1" ("SQL query") -> [w345]
    shift-right: [w341] -> w44
    shift-left: w43 -> [w344]
    shift-right: [w342] -> _
    shift-left: w42 -> [w343]
    shift-right: [w340] -> _
    shift-left: _ -> [w339]
    shift-right: [w337] -> _
    shift-left: _ -> [w338]
    tunnel: w33 -> [_]
    tunnel: w31 -> [_]
    shift-right: [w241] -> _
    shift-left: FALSE -> [w244]
    tunnel: w29 -> [_]
    stop <- w361 stop-if-true
    w203 = i32[] [100, 100, 100, 100, 100, 100, 100]
    w206 = TRUE
    w293 = 0 ("index (row)")
    w301 = i8 0
    w302 = 0.0
    w267 = 20
    # "charge"
    # "Empirical Delay Divisor"
    # "Mass"
    # "velocity"
    # "Sensitivity"
    # "Sampling Rate"
    # "Need to add Low and High mass"
    n153 = xnode "Invoke Method"("FPGA VI Reference In"=w367, "error in"=w366) -> ("FPGA VI Reference Out"=w261:refnum<k20>, "error out"=w260:errorcluster)  [unwired: 1 out]
    n154 = Bundle("Filter 1 Peak"=w353, "Filter 2 Peak"=w352, "Filter 3 Peak"=w351, "Filter 4 Peak"=w350, "Filter 5 Peak"=w349, "Filter 6 Peak"=w348, "Filter 7 Peak"=w347) -> (w333:T4)  [unwired: 1 in]
    n155 = call-poly <vilib>:"DB Tools Execute Query.vi"("error in (no error)"=w343, "SQL query"=w346, "connection reference"=w344) -> ("error out"=w321:errorcluster, "recordset reference"=w322:T5)  [unwired: 5 in]
    n156 = Wait (ms)(milliseconds to wait=u32 100) -> ()  [unwired: 1 out]
    n157 = local read "Delay Ring"() -> (w245:dbl)
    n158 = Unbundle By Name(w260) -> ("status"=w365:bool)
    n159 = call-poly <vilib>:"DB Tools Fetch Recordset Data.vi"("error in (no error)"=w321, "recordset reference"=w322) -> ("error out"=w299:errorcluster, "recordset data"=w312:variant[][], "recordset reference out"=w300:T5)  [unwired: 3 in]
    n160 = Equal?(x=w245, y=0.0) -> (x = y?=w246:bool)
    n161 = case shown="False" w246 {
      tunnel: [FALSE ("Add Delay") "Add Delay"] -> w264
      tunnel: w245 -> [w396 _]
      frame False {
        w397 = T2."Disabled and Grayed Out" ("Disabled")
        n162 = property on="Delay Value" class="DigNum (strict)"("DisabledEnum"=w397, "Value"=w396) -> ()  [unwired: 2 in, 2 out]
        n163 = property on="Add Delay" class="Bool (strict)"("DisabledEnum"=w397) -> ()  [unwired: 2 in, 2 out]
      }
      frame True {
        w398 = T2."Enabled" ("Disabled")
        n164 = property on="Delay Value" class="DigNum (strict)"("DisabledEnum"=w398) -> ()  [unwired: 2 in, 2 out]
        n165 = property on="Add Delay" class="Bool (strict)"("DisabledEnum"=w398) -> ()  [unwired: 2 in, 2 out]
      }
    }
    n166 = call-poly <vilib>:"DB Tools Free Object.vi"("error in (no error)"=w299, "recordset reference"=w300) -> ("error out"=w297:errorcluster, "connection reference"=w298:T3)  [unwired: 8 in]
    n167 = call-poly <vilib>:"DB Tools Execute Query.vi"("error in (no error)"=w297, "SQL query"=w345, "connection reference"=w298) -> ("error out"=w295:errorcluster, "recordset reference"=w296:T5)  [unwired: 5 in]
    n168 = Index Array(array=w312) -> (element=w311:variant[])  [unwired: 2 in]
    n169 = Or(x=w365, y="stop") -> (x .or. y?=w361:bool)
    "stopping" <- w361
    n170 = local read "Auto Threshold"() -> (w242:bool)
    n171 = call-poly <vilib>:"DB Tools Fetch Recordset Data.vi"("error in (no error)"=w295, "recordset reference"=w296) -> ("error out"=w268:errorcluster, "recordset data"=w294:variant[][], "recordset reference out"=w269:T5)  [unwired: 3 in]
    n172 = Index Array(array=w311, index #1=1 ("index"), index #2=2 ("index"), index #3=3 ("index"), index #4=4 ("index"), index #5=5 ("index"), index #6=6 ("index"), index #7=7 ("index"), index #8=8 ("index")) -> (element #1=w310:variant, element #2=w309:variant, element #3=w308:variant, element #4=w307:variant, element #5=w306:variant, element #6=w305:variant, element #7=w304:variant, element #8=w303:variant)
    n173 = case shown="True" w264 {
      frame False {
      }
      frame True {
        n174 = stacked-sequence {
          frame #0 {
            n175 = property on="Delay Ring" class="Ring (strict)"() -> ("StringsAndValues[]"=w402:T6)  [unwired: 2 in, 2 out]
            n176 = Bundle("Delay Name"="Delay Name", "Delay Value"="Delay Value") -> (w407:cluster{"Delay Name":string, "Delay Value":dbl})  [unwired: 1 in]
            n177 = Array Size(array=w402) -> (size(s)=w405:i32)
            n178 = for {
              tunnel: w402 -> [w412] mode=indexing
              tunnel: [w411] -> w401 mode=indexing
              n179 = Unbundle(w412) -> ("Value"=w411:dbl)  [unwired: 1 out]
            }
            n180 = Decrement(x=w405) -> (x-1=w404:i32)
            n181 = Search 1D Array(1D array=w401, element="Delay Value") -> (index of element=w409:i32)  [unwired: 1 in]
            n182 = Insert Into Array(array=w402, index=w404, new element=w407) -> (w406:T6)
            n183 = Equal?(x=w409, y=-1) -> (x = y?=w403:bool)
            n184 = case shown="True" w403 {
              tunnel: w406 -> [_ w421]
              frame False {
                n185 = One Button Dialog(message="Value Already Exists") -> ()  [unwired: 1 in, 1 out]
              }
              frame True {
                n186 = Array Size(array=w421) -> (size(s)=w423:i32)
                n187 = Decrement(x=w423) -> (x-1=w422:i32)
                n188 = call <userlib>:"Current VI's Path__ogtk.vi"() -> ("Current VI's Path (+ Relative)"=w427:path)  [unwired: 1 in]
                n189 = for {
                  N: w422 -> [_]
                  tunnel: w421 -> [w437] mode=indexing
                  tunnel: [w432] -> w424 mode=indexing
                  n190 = Unbundle(w437) -> ("String"=w433:string, "Value"=w436:dbl)
                  n191 = Format Into String(format string="%f", w436) -> (resulting string=w434:string)  [unwired: 2 in, 1 out]
                  n192 = Build Array(w433, w434) -> (w432:string[])
                }
                n193 = property on="Delay Ring" class="Ring (strict)"("StringsAndValues[]"=w421) -> ()  [unwired: 2 in, 2 out]
                n194 = Strip Path(path=w427) -> (stripped path=w415:path)  [unwired: 1 out]
                n195 = call-poly <userlib>:"Strip Path Extension__ogtk.vi"("path"=w415) -> ("extension"=w418:string)  [unwired: 1 out]
                n196 = Equal?(x="exe", y=w418) -> (x = y?=w416:bool)
                n197 = case shown="False" w416 {
                  tunnel: w415 -> [w429 w431]
                  tunnel: [w429 w430] -> w414
                  frame False {
                  }
                  frame True {
                    n198 = Strip Path(path=w431) -> (stripped path=w430:path)  [unwired: 1 out]
                  }
                }
                n199 = Array To Spreadsheet String(array=w424, 3:"%s" ("format string")) -> (spreadsheet string=w420:string)  [unwired: 1 in]
                n200 = Build Path(base path=w414, name or relative path="delay_ring.txt") -> (appended path=w425:path)
                n201 = call <vilib>:"Trim Whitespace.vi"("string"=w420) -> ("trimmed string"=w419:string)  [unwired: 1 in]
                n202 = Write to Text File(file (use dialog)=w425, text=w419) -> ()  [unwired: 2 in, 3 out]
              }
            }
          }
          frame #1 {
            n203 = property on="Add Delay" class="Bool (strict)"("Value"=FALSE ("Add Delay")) -> ()  [unwired: 2 in, 2 out]
          }
        }
      }
    }
    n204 = call-poly <vilib>:"DB Tools Free Object.vi"("error in (no error)"=w268, "recordset reference"=w269) -> ("error out"=w342:errorcluster, "connection reference"=w341:T3)  [unwired: 8 in]
    "error out" <- w342
    n205 = Index Array(array=w294, index (row)=w293, index (col)=w293) -> (element=w292:variant)
    n206 = Or(x=w242, y=w244) -> (x .or. y?=w243:bool)
    n207 = xnode "Read/Write Control"("FPGA VI Reference In"=w261, "error in"=w260, "One Shot"="One Shot Mode", "Reset One Shot"="Rearm Trigger") -> ("FPGA VI Reference Out"=w254:refnum<k20>, "error out"=w253:errorcluster)
    n208 = xnode "Database Variant To Data"("database variant"=w309, "type"=w302) -> ("data"=w217:dbl)  [unwired: 1 in, 1 out]
    n209 = xnode "Database Variant To Data"("database variant"=w310, "type"=w302) -> ("data"=w218:dbl)  [unwired: 1 in, 1 out]
    n210 = xnode "Database Variant To Data"("database variant"=w307, "type"=w302) -> ("data"=w216:dbl)  [unwired: 1 in, 1 out]
    n211 = xnode "Database Variant To Data"("database variant"=w308, "type"=w302) -> ("data"=w215:dbl)  [unwired: 1 in, 1 out]
    n212 = xnode "Database Variant To Data"("database variant"=w305, "type"=w302) -> ("data"=w214:dbl)  [unwired: 1 in, 1 out]
    n213 = xnode "Database Variant To Data"("database variant"=w306, "type"=w302) -> ("data"=w213:dbl)  [unwired: 1 in, 1 out]
    n214 = xnode "Database Variant To Data"("database variant"=w304, "type"=w301) -> ("data"=w286:i8)  [unwired: 1 in, 1 out]
    n215 = xnode "Database Variant To Data"("database variant"=w303, "type"=w301) -> ("data"=w285:i8)  [unwired: 1 in, 1 out]
    n216 = Build Array(w217, w218) -> (w289:dbl[])
    n217 = xnode "Database Variant To Data"("database variant"=w292, "type"=0.0) -> ("data"=w212:dbl)  [unwired: 1 in, 1 out]
    "Peletron (MV)" <- w212
    n218 = Build Array(w216, w215) -> (w288:dbl[])
    n219 = Build Array(w214, w213) -> (w287:dbl[])
    n220 = Equal To 0?(x="Delay Ring") -> (x = 0?=w211:bool)
    n221 = xnode "Read/Write Control"("FPGA VI Reference In"=w254, "error in"=w253) -> ("Not Armed?"=w252:bool, "Del Not Armed?"=w205:bool)  [unwired: 2 out]
    n222 = local read "Delay Value"() -> (w210:dbl)
    n223 = call "calc_variables.vi"("var2"=w285, "Peletron"=w212, "var1"=w286, "Mass"=w287, "Charge"=w288, "Velocity"=w289) -> ("Mass out"=w278:dbl[], "Charge out"=w281:dbl[], "Velocity out"=w284:dbl[])  [unwired: 3 in]
    n224 = property on="Rearm Trigger" class="Bool (strict)"(error in=w253, "Value"=FALSE ("Rearm Trigger")) -> ()  [unwired: 1 in, 2 out]
    n225 = Divide(x="Delay Ring", y=0.93) -> (x/y=w250:dbl)
    n226 = Select(t=w210, s=w211, f=w250) -> (s? t:f=w249:dbl)
    n227 = Not(x=w252) -> (.not. x?=→"Armed":bool)
    n228 = Not(x=w205) -> (.not. x?=→"Del Armed":bool)
    n229 = And(x=w211, y=w206) -> (x .and. y?=w207:bool)
    n230 = property on="Peletron (MV)" class="DigNum (strict)"() -> ("Value"=w290:dbl)  [unwired: 2 in, 2 out]
    n231 = case shown="True" w207 {
      selector: w207 -> [w368 _]
      tunnel: w210 -> [_ w370]
      tunnel: [w368 w369] -> w208
      frame False {
      }
      frame True {
        n232 = call-poly <userlib>:"Data Changed__ogtk.vi"("DBL"=w370) -> ("Changed"=w369:bool)
      }
    }
    n233 = To Fixed-Point(number=w249) -> (fixed-point=w263:fxp<+,16,7>)  [unwired: 1 in]
    n234 = Index Array(array=w281, index #1=0 ("index"), index #2=1 ("index")) -> (element #1=w273:dbl, element #2=w272:dbl)
    "High Charge Limit (fC)" <- w272
    "Low Charge Limit (fC)" <- w273
    n235 = Index Array(array=w284, index #1=0 ("index"), index #2=1 ("index")) -> (element #1=w275:dbl, element #2=w274:dbl)
    "High Velocity" <- w274
    "Low Velocity" <- w275
    n236 = Index Array(array=w278, index #1=0 ("index"), index #2=1 ("index")) -> (element #1=w271:dbl, element #2=w270:dbl)
    "Low Mass (kg)" <- w271
    "High Mass (kg)" <- w270
    n237 = Bundle("Numeric"=w275, "Numeric"=w274, "Numeric"=w273, "Numeric"=w272, "Numeric"=w271, "Numeric"=w270, w267, 26666666.59375, "Value"=w290, w263, w206) -> (w332:T7)  [unwired: 1 in]
    n238 = call "process_limits.vi"("old output cluster"=w339, "Input cluster"=w332) -> ("Update FPGA"=w266:bool, "output cluster"=w340:T8)  [unwired: 8 in]
    n239 = Unbundle By Name(w340) -> ("Low Velocity Count"=w328:i32, "High Velocity Count"=w327:i32, "Low Charge Limit (ADC ticks)"=w325:i16, "High Charge Limit (ADC ticks)"=w326:i16, "Low Mass (ADC*cycle^2)"=w330:i64, "High Mass (ADC*cycle^2)"=w331:i64, "Mult"=w262:fxp<+,16,7>)
    "Low velocity count" <- w328
    "High velocity count" <- w327
    "High Charge Limit" <- w326
    "Low Charge Limit" <- w325
    "High Mass Limit" <- w331
    "Low Mass Limit" <- w330
    n240 = Or(x=w266, y=w243) -> (x .or. y?=w248:bool)
    n241 = Or(x="Raise Threshold", y="Lower Threshold") -> (x .or. y?=w219:bool)
    n242 = Or(x=w219, y=w248) -> (x .or. y?=w220:bool)
    n243 = Build Array("Filter1 Threshold", "Filter2 Threshold", "Filter3 Threshold", "Filter4 Threshold", "Filter5 Threshold", "Filter6 Threshold", "Filter7 Threshold") -> (w202:i32[])
    n244 = case shown="True" "Lower Threshold" {
      tunnel: w202 -> [w371 w382]
      tunnel: w203 -> [_ w381]
      tunnel: [w371 w372] -> w233
      frame False {
      }
      frame True {
        n245 = Add(x=w382, y=w381) -> (x+y=w372:i32[])
        n246 = local write "Lower Threshold"(FALSE ("Lower Threshold")) -> ()
        n247 = Index Array(array=w372) -> (element #1=w379:i32, element #2=w378:i32, element #3=w377:i32, element #4=w376:i32, element #5=w375:i32, element #6=w374:i32, element #7=w373:i32)  [unwired: 7 in]
        n248 = local write "Filter1 Threshold"(w379) -> ()
        n249 = local write "Filter2 Threshold"(w378) -> ()
        n250 = local write "Filter3 Threshold"(w377) -> ()
        n251 = local write "Filter4 Threshold"(w376) -> ()
        n252 = local write "Filter5 Threshold"(w375) -> ()
        n253 = local write "Filter6 Threshold"(w374) -> ()
        n254 = local write "Filter7 Threshold"(w373) -> ()
      }
    }
    n255 = Or(x=w220, y=w208) -> (x .or. y?=w209:bool)
    "Updating FPGA" <- w209
    n256 = case shown="True" "Raise Threshold" {
      tunnel: w202 -> [_ w393]
      tunnel: w203 -> [_ w383]
      frame False {
      }
      frame True {
        n257 = Subtract(x=w393, y=w383) -> (x-y=w384:i32[])
        n258 = local write "Raise Threshold"(FALSE ("Raise Threshold")) -> ()
        n259 = Index Array(array=w384) -> (element #1=w391:i32, element #2=w390:i32, element #3=w389:i32, element #4=w388:i32, element #5=w387:i32, element #6=w386:i32, element #7=w385:i32)  [unwired: 7 in]
        n260 = local write "Filter1 Threshold"(w391) -> ()
        n261 = local write "Filter2 Threshold"(w390) -> ()
        n262 = local write "Filter3 Threshold"(w389) -> ()
        n263 = local write "Filter4 Threshold"(w388) -> ()
        n264 = local write "Filter5 Threshold"(w387) -> ()
        n265 = local write "Filter6 Threshold"(w386) -> ()
        n266 = local write "Filter7 Threshold"(w385) -> ()
      }
    }
    n267 = Index Array(array=w233) -> (element #1=w236:i32, element #2=w234:i32, element #3=w231:i32, element #4=w229:i32, element #5=w227:i32, element #6=w225:i32, element #7=w223:i32)  [unwired: 7 in]
    n268 = case shown="True" w209 {
      tunnel: w261 -> [w440 w468]
      tunnel: w260 -> [w441 w467]
      tunnel: [w440 w466] -> w363
      tunnel: [w441 w465] -> w362
      tunnel: w236 -> [_ w464]
      tunnel: w234 -> [_ w463]
      tunnel: w231 -> [_ w462]
      tunnel: w229 -> [_ w461]
      tunnel: w227 -> [_ w460]
      tunnel: w225 -> [_ w459]
      tunnel: w223 -> [_ w458]
      tunnel: [w439 w444] -> w337
      tunnel: w331 -> [_ w450]
      tunnel: w330 -> [_ w449]
      tunnel: w328 -> [_ w448]
      tunnel: w327 -> [_ w447]
      tunnel: w326 -> [_ w446]
      tunnel: w325 -> [_ w445]
      tunnel: w338 -> [w439 _]
      tunnel: w262 -> [_ w442]
      frame False {
      }
      frame True {
        n269 = xnode "Read/Write Control"("FPGA VI Reference In"=w468, "error in"=w467, "Low Velocity Count"=w448, "High Velocity Count"=w447, "Filter 1 threshold"=w464, "Filter 2 threshold"=w463, "Filter 3 threshold"=w462, "Filter 4 threshold"=w461, "Filter 5 threshold"=w460, "Filter 6 threshold"=w459, "Filter 7 threshold"=w458, "High Charge Limit"=w446, "Low Charge Limit"=w445, "High Mass Limit"=w450, "Low Mass Limit"=w449, "Mult1"=w442) -> ("FPGA VI Reference Out"=w466:refnum<k20>, "error out"=w465:errorcluster, "Filter 1 Detector 3 Correlation"=w457:i32, "Filter 2 Detector 3 Correlation"=w456:i32, "Filter 3 Detector 3 Correlation"=w455:i32, "Filter 4 Detector 3 Correlation"=w454:i32, "Filter 5 Detector 3 Correlation"=w453:i32, "Filter 6 Detector 3 Correlation"=w452:i32, "Filter 7 Detector 3 Correlation"=w451:i32)
        n270 = Get Date/Time In Seconds() -> (seconds since 1Jan1904=→"Last Update:":timestamp)
        n271 = Bundle("Filter 1 Detector 3 Correlation"=w457, "Filter 2 Detector 3 Correlation"=w456, "Filter 3 Detector 3 Correlation"=w455, "Filter 4 Detector 3 Correlation"=w454, "Filter 5 Detector 3 Correlation"=w453, "Filter 6 Detector 3 Correlation"=w452, "Filter 7 Detector 3 Correlation"=w451) -> (w444:T9)  [unwired: 1 in]
      }
    }
    n272 = call "filter_peaks.vi"("Correlation cluster"=w337, "Filter peak cluster"=w333, "Zero out"="Zero Peak Values", "Run Mode"="Run Mode") -> ("Blinking"=w324:bool, "status"=w329:T2, "Filter peak output"=w334:T4)  [unwired: 5 in]
    n273 = shared-variable "My Computer\\Network Shared Variables.lvlib\\FPGA Trigger"() -> ()  [unwired: 1 in, 2 out]
    n274 = Unbundle By Name(w334) -> ("Filter 1 Peak"=w360:i32, "Filter 2 Peak"=w359:i32, "Filter 3 Peak"=w358:i32, "Filter 4 Peak"=w357:i32, "Filter 5 Peak"=w356:i32, "Filter 6 Peak"=w355:i32, "Filter 7 Peak"=w354:i32)
    "Filter 1 Peak" <- w360
    "Filter 2 Peak" <- w359
    "Filter 3 Peak" <- w358
    "Filter 4 Peak" <- w357
    "Filter 5 Peak" <- w356
    "Filter 6 Peak" <- w355
    "Filter 7 Peak" <- w354
    n275 = property on="Filter 3 Peak" class="DigNum (strict)"("DisabledEnum"=w329, "Blinking"=w324) -> ()  [unwired: 2 in, 2 out]
    n276 = property on="Filter 4 Peak" class="DigNum (strict)"("DisabledEnum"=w329, "Blinking"=w324) -> ()  [unwired: 2 in, 2 out]
    n277 = property on="Filter 7 Peak" class="DigNum (strict)"("DisabledEnum"=w329, "Blinking"=w324) -> ()  [unwired: 2 in, 2 out]
    n278 = property on="Filter 5 Peak" class="DigNum (strict)"("DisabledEnum"=w329, "Blinking"=w324) -> ()  [unwired: 2 in, 2 out]
    n279 = property on="Filter 6 Peak" class="DigNum (strict)"("DisabledEnum"=w329, "Blinking"=w324) -> ()  [unwired: 2 in, 2 out]
    n280 = property on="Filter 2 Peak" class="DigNum (strict)"("DisabledEnum"=w329, "Blinking"=w324) -> ()  [unwired: 2 in, 2 out]
    n281 = property on="Filter 1 Peak" class="DigNum (strict)"("DisabledEnum"=w329, "Blinking"=w324) -> ()  [unwired: 2 in, 2 out]
    n282 = local read "Update Threshold"() -> (w239:bool)
    n283 = call-poly <userlib>:"Data Changed__ogtk.vi"("Boolean"=w239) -> ("Changed"=w240:bool)
    n284 = And(x=w240, y=w239) -> (x .and. y?=w238:bool)
    n285 = case shown="True" w238 {
      frame False {
      }
      frame True {
        n286 = local write "Update Threshold"(FALSE ("Update Threshold")) -> ()
      }
    }
    n287 = Or(x=w242, y=w239) -> (x .or. y?=w241:bool)
    "Sensitivity" <- w267
  }
  n288 = while {
    stop <- w758 stop-if-true
    n289 = case shown="False" "Rate Limiting" {
      frame False {
        n290 = property on="Rearm Trigger" class="Bool (strict)"("DisabledEnum"=T2."Enabled" ("Disabled")) -> ()  [unwired: 2 in, 2 out]
        n291 = property on="One Shot Mode" class="Bool (strict)"("DisabledEnum"=T2."Enabled" ("Disabled")) -> ()  [unwired: 2 in, 2 out]
      }
      frame True {
        n292 = local read "Armed"() -> (w762:bool)
        n293 = Get Date/Time In Seconds() -> (seconds since 1Jan1904=w761:timestamp)
        n294 = property on="Rearm Trigger" class="Bool (strict)"("DisabledEnum"=T2."Disabled and Grayed Out" ("Disabled")) -> ()  [unwired: 2 in, 2 out]
        n295 = case shown="False" w762 {
          tunnel: [w769 FALSE] -> w766
          tunnel: w761 -> [w768 _]
          frame False {
            n296 = flat-sequence {
              tunnel: w768 -> [w770]
              tunnel: [w770] -> w767
              tunnel: [TRUE] -> w769
              tunnel: w767 -> [w776]
              frame #0 {
                n297 = Multiply(x="Min. Time\nBetween Shots (s)", y=1000.0) -> (x*y=w773:dbl)
                n298 = Round Toward +Infinity(x=w773) -> (ceil(x): smallest int >= x=w771:dbl)
                n299 = Wait (ms)(milliseconds to wait=w771) -> ()  [unwired: 1 out]
              }
              frame #1 {
                n300 = Get Date/Time In Seconds() -> (seconds since 1Jan1904=w777:timestamp)
                n301 = Subtract(x=w777, y=w776) -> (x-y=→"Time Betwee Shots":dbl)
              }
            }
          }
          frame True {
          }
        }
        n302 = property on="One Shot Mode" class="Bool (strict)"("DisabledEnum"=T2."Disabled and Grayed Out" ("Disabled"), "Value"=TRUE ("One Shot Mode")) -> ()  [unwired: 2 in, 2 out]
        n303 = local write "Rearm Trigger"(w766) -> ()
      }
    }
    n304 = property on="stopping" class="Bool (strict)"() -> ("Value"=w758:bool)  [unwired: 2 in, 2 out]
  }
  n305 = call "connect out.vi"("error in (no error)"=w42, "connection reference"=w44) -> ()  [unwired: 9 in, 1 out]
  n306 = xnode "Close FPGA VI Reference"("FPGA VI Reference In"=w68, "error in"=w67) -> ("error out"=w70:errorcluster)
  n307 = call <vilib>:"General Error Handler.vi"("error in (no error)"=w70) -> ()  [unwired: 10 in, 5 out]
